vi "Word_Create_Document.vi"(4 "error in":errorcluster, 6 "Template Path":path, 7 "word application":refnum<k7>) -> (0 "error out":errorcluster, 3 "references":T1)   [LabVIEW 2020, in "NI_ReportGenerationToolkit.lvlib"]
uses:
  <vilib>/addons/_office/NI_ReportGenerationToolkit.lvlib
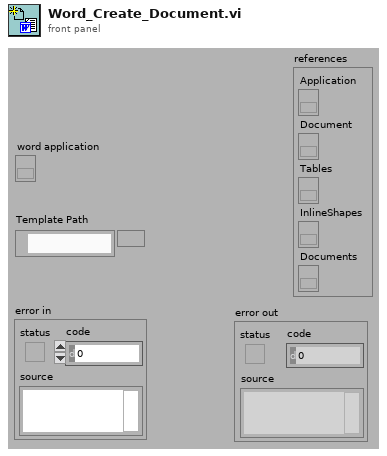
[diagram p1: front panel]
types:
  T1 = cluster{"Application":refnum<k7>, "Document":refnum<k7>, "Tables":refnum<k7>, "InlineShapes":refnum<k7>, "Documents":refnum<k7>}
  T2 = cluster{"word application":refnum<k7>, "Add":refnum<k7>, "Tables":refnum<k7>, "InlineShapes":refnum<k7>, "Documents":refnum<k7>}
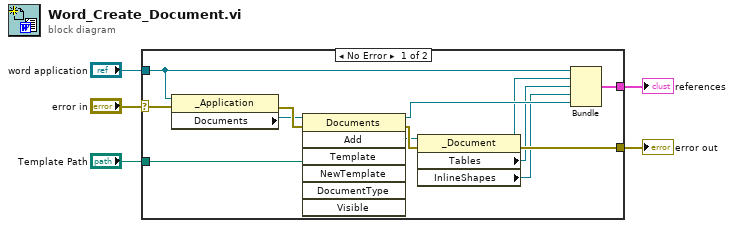
[diagram p0: block diagram]
diagram:
  n1 = case shown="No Error" "error in" {
    selector: "error in" -> [w6 w19]
    tunnel: [w16 w19] -> w5
    tunnel: "Template Path" -> [w14 _]
    tunnel: [w11 _] -> w3
    tunnel: "word application" -> [w7 _]
    frame No Error {
      n2 = property class="_Application"(reference=w7, error in=w6) -> (error out=w18:errorcluster, "Documents"=w17:refnum<k7>)  [unwired: 1 out]
      n3 = invoke class="Documents" method="Add"(reference=w17, error in=w18, "Template"=w14) -> (reference out=w15:refnum<k7>, error out=w9:errorcluster, "Add"=w8:refnum<k7>)  [unwired: 4 in, 4 out]
      n4 = property class="_Document"(reference=w8, error in=w9) -> (reference out=w10:refnum<k7>, error out=w16:errorcluster, "Tables"=w13:refnum<k7>, "InlineShapes"=w12:refnum<k7>)
      n5 = Bundle("word application"=w7, "Add"=w10, "Tables"=w13, "InlineShapes"=w12, "Documents"=w15) -> (w11:T2)  [unwired: 1 out]
    }
    frame Error {
    }
  }
  "error out" <- w5
  "references" <- w3
